vi "Resize Headers.vi"(8 "error in":errorcluster, 10 "Total Size":dbl, 11 "Column Headers":string[](array[string])) -> (0 "error out":errorcluster, 2 "Auto width":bool, 3 "Resized":dbl[](array[numeric]) format="%.3g")   [LabVIEW 2020]
panel:
  out "sum":dbl
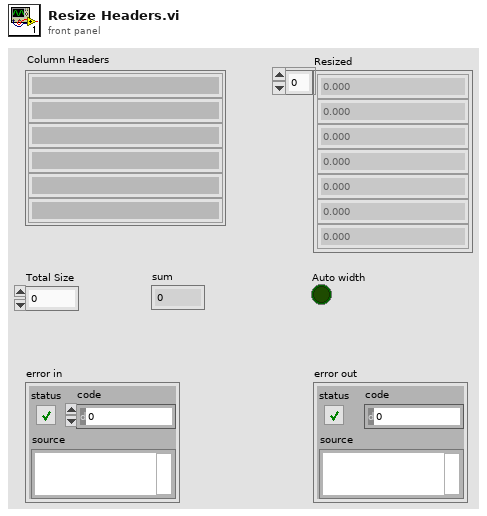
[diagram p1: front panel]
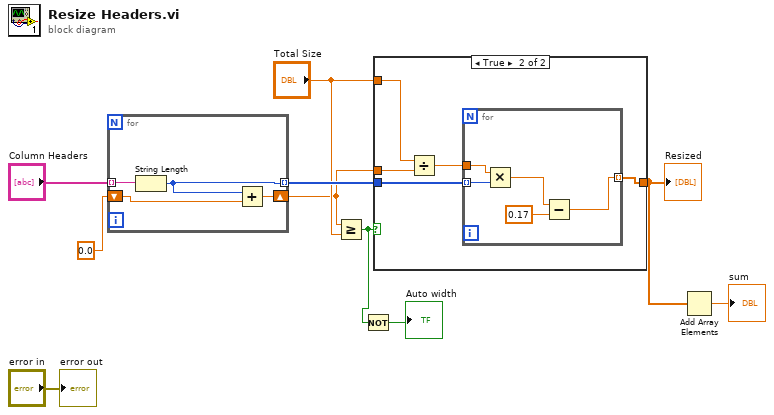
[diagram p0: block diagram]
diagram:
  n1 = for {
    tunnel: "Column Headers" -> [w14] mode=indexing
    tunnel: [w11] -> w8 mode=indexing
    shift-right: [w13] -> w6
    shift-left: 0.0 -> [w12]
    n2 = String Length(string=w14) -> (length=w11:i32)
    n3 = Add(x=w11, y=w12) -> (x+y=w13:dbl)
  }
  n4 = Greater Or Equal?(x=w6, y="Total Size") -> (x >= y?=w3:bool)
  n5 = Not(x=w3) -> (.not. x?=→"Auto width":bool)
  n6 = case shown="True" w3 {
    tunnel: w8 -> [w15 w17]
    tunnel: [w15 w16] -> w2
    tunnel: "Total Size" -> [_ w20]
    tunnel: w6 -> [_ w19]
    frame False {
    }
    frame True {
      n7 = Divide(x=w20, y=w19) -> (x/y=w18:dbl)
      n8 = for {
        tunnel: w18 -> [w25]
        tunnel: w17 -> [w24] mode=indexing
        tunnel: [w21] -> w16 mode=indexing
        n9 = Multiply(x=w25, y=w24) -> (x*y=w23:dbl)
        n10 = Subtract(x=w23, y=0.17) -> (x-y=w21:dbl)
      }
    }
  }
  "Resized" <- w2
  n11 = Add Array Elements(numeric array=w2) -> (sum=→"sum":dbl)
  "error out" <- "error in"
